vi "UVflourescence.vi"() -> ()   [LabVIEW 2009]
uses:
  <vilib>/DAQmx/write.llb/DAQmx Write (Digital Wfm 1Chan NSamp).vi
  <vilib>/DAQmx/configure/timing.llb/DAQmx Timing (Sample Clock).vi
  <vilib>/DAQmx/create/channels.llb/DAQmx Create Channel (DO-Digital Output).vi
  <vilib>/DAQmx/configure/timing.llb/DAQmx Timing (Implicit).vi
  <vilib>/DAQmx/create/channels.llb/DAQmx Create Channel (CO-Pulse Generation-Frequency).vi
  <vilib>/DAQmx/create/channels.llb/DAQmx Create Channel (CI-Count Edges).vi
  <vilib>/Waveform/DWDTOps.llb/DWDT Digital Size.vi
  <vilib>/DAQmx/read.llb/DAQmx Read (Counter 1D U32 1Chan NSamp).vi
  Program Files/National Instruments/LabVIEW 2009/resource/objmgr/daqmx.rc
  <vilib>/Analysis/NI_AALBase.lvlib
panel:
  out "Mean/Variance":dbl
  out "Variance":dbl format="%0.2f"
  out "Mean":dbl format="%0.2f"
  out "PMT Counts":cluster{"mean":dbl, u32}(graph)
  in  "Samples per block":i32=100 min=1 step=1
  out "x = 0?":bool
  out "Waveform Graph":u32[](graph)
  in  "Stop":bool
  in  "Sample Time":dbl=5e-07
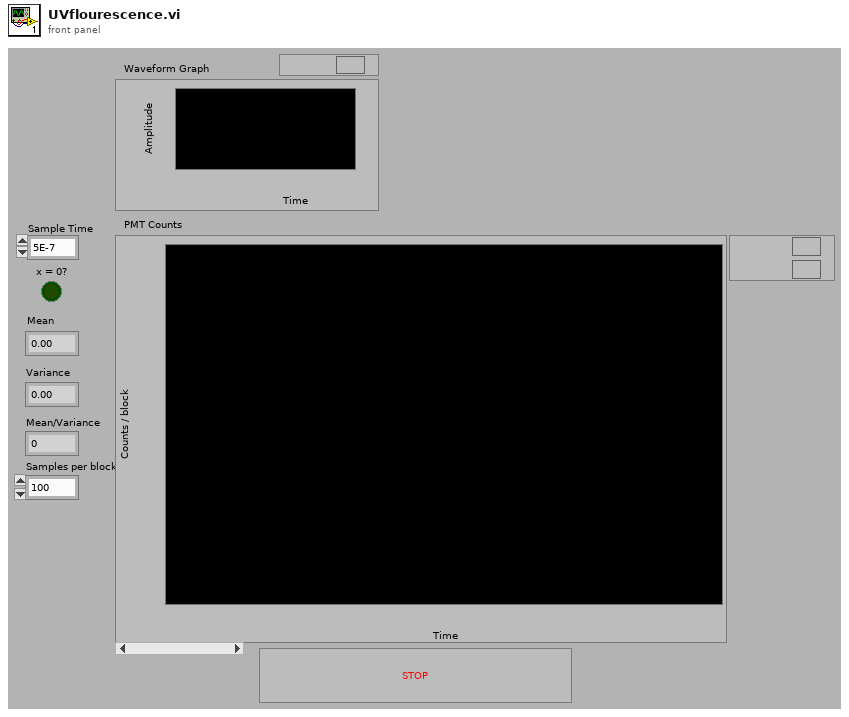
[diagram p1: front panel]
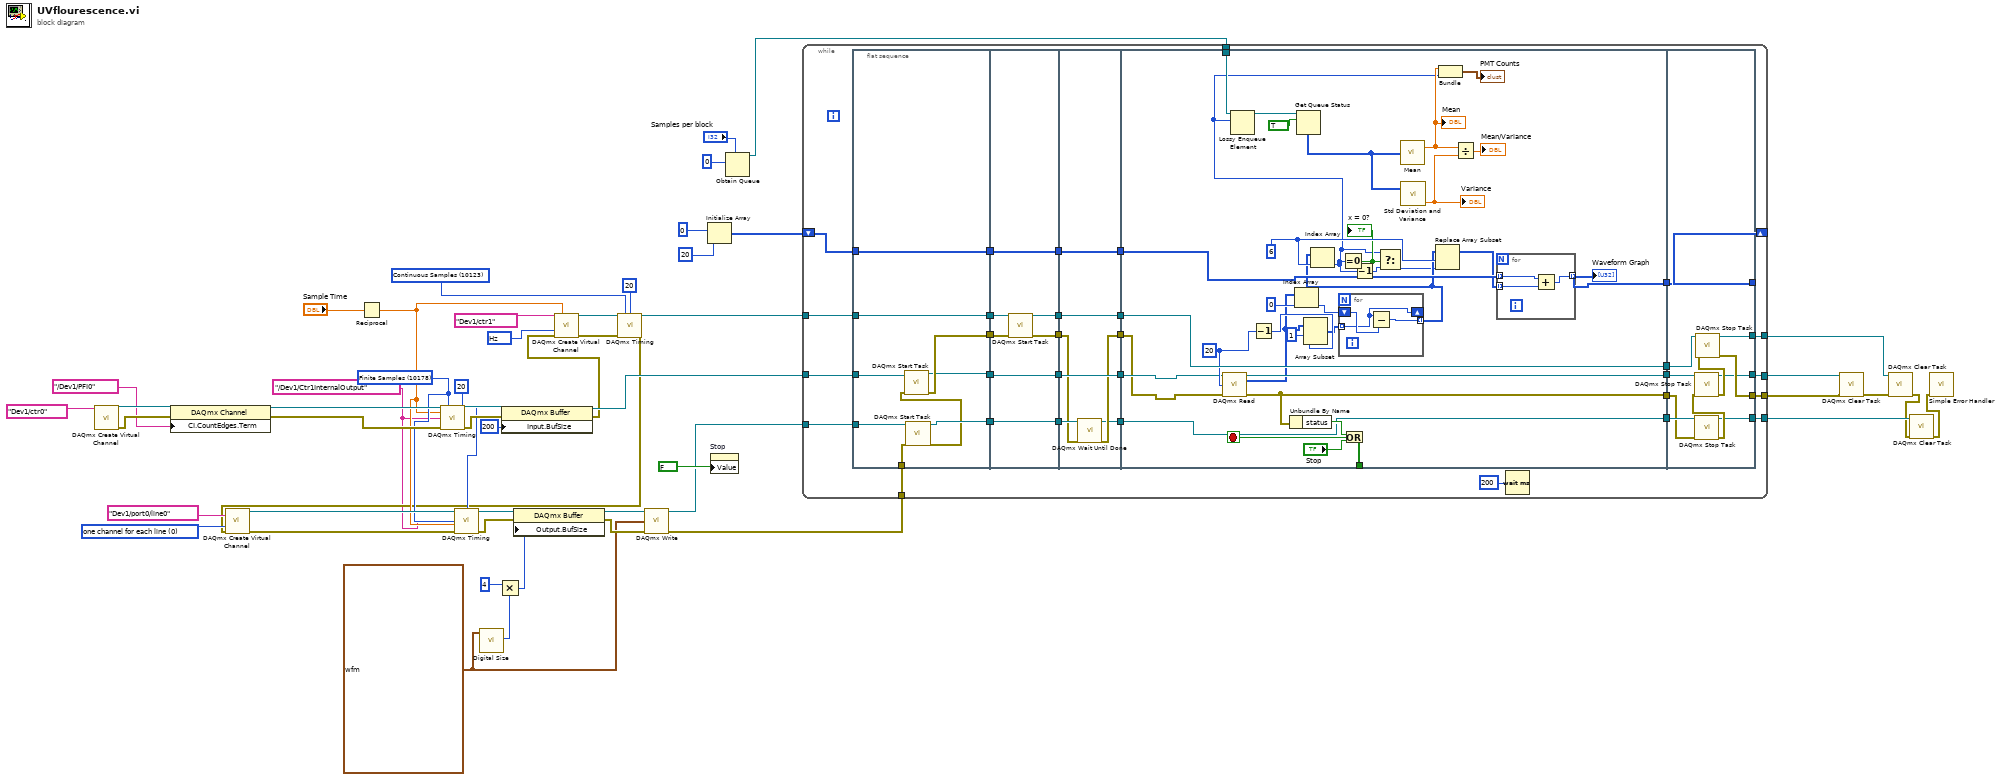
[diagram p0: block diagram]
diagram:
  w19 = digitalwaveform {"t0"=timestamp(0 s since 1904-01-01), "dt"=1e-06, "Y"={"transitions"=[], "data"=[[1], [1], [1], [1], [0], [0], [0], [0], [0], [1], [1], [1], [1], [0], [0], [0], [0], [0], [0], [0]]}, "error"={"status"=FALSE, "code"=37421928, "source"=""}} ("data")
  w24 = 0 items=["one channel for each line", "one channel for all lines"] ("line grouping")
  w14 = 10178 items=["Finite Samples"=10178, "Continuous Samples"=10123, "Hardware Timed Single Point"=12522] ("sample mode")
  w15 = 20 ("samples per channel")
  w4 = tag "/Dev1/Ctr1InternalOutput" ("source")
  w50 = 10373 items=["Hz"=10373] ("units")
  w42 = 10123 items=["Finite Samples"=10178, "Continuous Samples"=10123, "Hardware Timed Single Point"=12522] ("sample mode")
  n1 = call-poly <vilib>:"DAQmx Create Virtual Channel.vi"("counter"=tag "Dev1/ctr0") -> ("task out"=w47:refnum<k21>, "error out"=w46:errorcluster)  [unwired: 13 in]
  n2 = property class="DAQmx Channel"(reference=w47, error in=w46, "CI.CountEdges.Term"=tag "/Dev1/PFI0") -> (reference out=w37:refnum<k21>, error out=w38:errorcluster)
  n3 = Reciprocal(x="Sample Time") -> (1/x=w13:dbl)
  n4 = call-poly <vilib>:"DAQmx Timing.vi"("task/channels in"=w37, "sample mode"=w14, "samples per channel"=w15, "rate"=w13, "source"=w4, "error in"=w38) -> ("task out"=w31:refnum<k21>, "error out"=w30:errorcluster)  [unwired: 8 in]
  n5 = call-poly <vilib>:"Digital Size.vi"("digital waveform in"=w19) -> ("number of samples"=w18:i32)  [unwired: 7 in, 3 out]
  n6 = Multiply(x=4, y=w18) -> (x*y=w16:i32)
  n7 = property class="DAQmx Buffer"(reference=w31, error in=w30, "Input.BufSize"=u32 200) -> (reference out=w29:refnum<k21>, error out=w28:errorcluster)
  n8 = call-poly <vilib>:"DAQmx Create Virtual Channel.vi"("frequency"=w13, "counter"=tag "Dev1/ctr1", "units"=w50, "error in"=w28) -> ("task out"=w49:refnum<k21>, "error out"=w48:errorcluster)  [unwired: 10 in]
  n9 = call-poly <vilib>:"DAQmx Timing.vi"("task/channels in"=w49, "sample mode"=w42, "samples per channel"=20, "error in"=w48) -> ("task out"=w11:refnum<k21>, "error out"=w8:errorcluster)  [unwired: 10 in]
  n10 = call-poly <vilib>:"DAQmx Create Virtual Channel.vi"("lines"=tag "Dev1/port0/line0", "line grouping"=w24, "error in"=w8) -> ("task out"=w26:refnum<k21>, "error out"=w25:errorcluster)  [unwired: 11 in]
  n11 = call-poly <vilib>:"DAQmx Timing.vi"("task/channels in"=w26, "sample mode"=w14, "samples per channel"=w15, "rate"=w13, "source"=w4, "error in"=w25) -> ("task out"=w22:refnum<k21>, "error out"=w21:errorcluster)  [unwired: 8 in]
  n12 = property class="DAQmx Buffer"(reference=w22, error in=w21, "Output.BufSize"=w16) -> (reference out=w12:refnum<k21>, error out=w20:errorcluster)
  n13 = call-poly <vilib>:"DAQmx Write.vi"("task/channels in"=w12, "data"=w19, "error in"=w20) -> ("task out"=w10:refnum<k21>, "error out"=w9:errorcluster)  [unwired: 10 in, 1 out]
  n14 = Initialize Array(0, 20 ("dimension size")) -> (w39:i32[])
  n15 = property on="Stop" class="Bool (strict)"("Value"=FALSE) -> ()  [unwired: 2 in, 2 out]
  n16 = Obtain Queue(max queue size (-1, unlimited)="Samples per block", element data type=u32 0) -> (queue out=w1:refnum<queue>)  [unwired: 3 in, 2 out]
  n17 = while {
    tunnel: [w81] -> w34
    tunnel: [w82] -> w35
    tunnel: w29 -> [w83]
    shift-right: [w75] -> _
    shift-left: w39 -> [w84]
    tunnel: w11 -> [w80]
    tunnel: [w70] -> w33
    tunnel: w10 -> [w69]
    tunnel: w9 -> [w68]
    tunnel: [w55] -> w7
    tunnel: w1 -> [w53]
    stop <- w85 stop-if-true
    n18 = flat-sequence {
      tunnel: w80 -> [w93]
      tunnel: w83 -> [w92]
      tunnel: w84 -> [w94]
      tunnel: [w94] -> w79
      tunnel: [w90] -> w78
      tunnel: [w93] -> w77
      tunnel: [w91] -> w76
      tunnel: w69 -> [w89]
      tunnel: w68 -> [w88]
      tunnel: [w87] -> w58
      tunnel: [w101] -> w67
      tunnel: [w100] -> w65
      tunnel: w79 -> [w101]
      tunnel: w78 -> [w100]
      tunnel: w77 -> [w99]
      tunnel: w76 -> [w98]
      tunnel: [w97] -> w63
      tunnel: [w96] -> w61
      tunnel: [w95] -> w59
      tunnel: w58 -> [w95]
      tunnel: w67 -> [w108]
      tunnel: [w108] -> w66
      tunnel: w65 -> [w107]
      tunnel: [w107] -> w64
      tunnel: w63 -> [w106]
      tunnel: [w106] -> w62
      tunnel: w61 -> [w104]
      tunnel: [w103] -> w60
      tunnel: w59 -> [w105]
      tunnel: [w102] -> w56
      tunnel: [w141] -> w85
      tunnel: w66 -> [w128]
      tunnel: w64 -> [w126]
      tunnel: [w137] -> w74
      tunnel: [w136] -> w73
      tunnel: [w127] -> w72
      tunnel: [w138] -> w71
      tunnel: w62 -> [w138]
      tunnel: w60 -> [w125]
      tunnel: [w124] -> w57
      tunnel: w56 -> [w124]
      tunnel: w53 -> [w110]
      tunnel: [w158] -> w75
      tunnel: [w154] -> w81
      tunnel: [w153] -> w82
      tunnel: w74 -> [w156]
      tunnel: w73 -> [w150]
      tunnel: w72 -> [w158]
      tunnel: w71 -> [w157]
      tunnel: [w152] -> w70
      tunnel: w57 -> [w151]
      tunnel: [w148] -> w55
      frame #0 {
        n19 = call <vilib>:"DAQmx Start Task.vi"("task/channels in"=w89, "error in"=w88) -> ("task out"=w87:refnum<k21>, "error out"=w86:errorcluster)  [unwired: 12 in]
        n20 = call <vilib>:"DAQmx Start Task.vi"("task/channels in"=w92, "error in"=w86) -> ("task out"=w90:refnum<k21>, "error out"=w91:errorcluster)  [unwired: 12 in]
      }
      frame #1 {
        n21 = call <vilib>:"DAQmx Start Task.vi"("task/channels in"=w99, "error in"=w98) -> ("task out"=w97:refnum<k21>, "error out"=w96:errorcluster)  [unwired: 12 in]
      }
      frame #2 {
        n22 = call <vilib>:"DAQmx Wait Until Done.vi"("task/channels in"=w105, "error in"=w104) -> ("task out"=w102:refnum<k21>, "error out"=w103:errorcluster)  [unwired: 12 in]
      }
      frame #3 {
        w123 = 6 ("index")
        w130 = 20 ("number of samples per channel")
        n23 = call-poly <vilib>:"DAQmx Read.vi"("task/channels in"=w126, "number of samples per channel"=w130, "error in"=w125) -> ("task out"=w137:refnum<k21>, "data"=w129:u32[], "error out"=w136:errorcluster)  [unwired: 10 in]
        n24 = Decrement(x=w130) -> (x-1=w132:i32)
        n25 = Unbundle By Name(w136) -> ("status"=w140:bool)
        n26 = Index Array(array=w129, index=0) -> (element=w134:u32)
        n27 = Array Subset(array=w129, index=1, length=w132) -> (w131:u32[])
        n28 = for {
          tunnel: [w147] -> w122 mode=indexing
          shift-right: [w145] -> _
          shift-left: w134 -> [w146]
          tunnel: w131 -> [w145] mode=indexing
          n29 = Subtract(x=w145, y=w146) -> (x-y=w147:u32)
        }
        n30 = Index Array(array=w122, index=w123) -> (element=w109:u32)
        n31 = Lossy Enqueue Element(queue=w110, element=w109) -> (queue out=w117:refnum<queue>)  [unwired: 1 in, 3 out]
        n32 = Get Queue Status(queue=w117, return elements? (F)=TRUE) -> (elements=w115:u32[])  [unwired: 1 in, 7 out]
        n33 = Equal To 0?(x=w109) -> (x = 0?=w120:bool)
        "x = 0?" <- w120
        n34 = Or(x=w140, y="Stop") -> (x .or. y?=w141:bool)
        n35 = Decrement(x=w109) -> (x-1=w119:u32)
        n36 = Select(t=w109, s=w120, f=w119) -> (s? t:f=w118:u32)
        n37 = call <vilib>:"Mean.vi"("X"=w115) -> ("mean"=w111:dbl)  [unwired: 1 out]
        "Mean" <- w111
        n38 = call <vilib>:"Std Deviation and Variance.vi"("X"=w115) -> ("variance"=w114:dbl)  [unwired: 1 in, 2 out]
        "Variance" <- w114
        n39 = Replace Array Subset(array=w122, new element=w118, index=w123) -> (w121:u32[])
        n40 = Bundle("mean"=w111, w109) -> (→"PMT Counts":cluster{"mean":dbl, u32})  [unwired: 1 in]
        n41 = Divide(x=w111, y=w114) -> (x/y=→"Mean/Variance":dbl)
        n42 = for {
          tunnel: w128 -> [w144] mode=indexing
          tunnel: w121 -> [w143] mode=indexing
          tunnel: [w142] -> w127 mode=indexing
          n43 = Add(x=w144, y=w143) -> (x+y=w142:u32)
        }
        "Waveform Graph" <- w127
      }
      frame #4 {
        n44 = call <vilib>:"DAQmx Stop Task.vi"("task/channels in"=w151, "error in"=w150) -> ("task out"=w148:refnum<k21>, "error out"=w149:errorcluster)  [unwired: 12 in]
        n45 = call <vilib>:"DAQmx Stop Task.vi"("task/channels in"=w156, "error in"=w149) -> ("task out"=w153:refnum<k21>, "error out"=w155:errorcluster)  [unwired: 12 in]
        n46 = call <vilib>:"DAQmx Stop Task.vi"("task/channels in"=w157, "error in"=w155) -> ("task out"=w152:refnum<k21>, "error out"=w154:errorcluster)  [unwired: 12 in]
      }
    }
    n47 = Wait (ms)(milliseconds to wait=u32 200) -> ()  [unwired: 1 out]
  }
  n48 = call <vilib>:"DAQmx Clear Task.vi"("task in"=w35, "error in"=w34) -> ("error out"=w44:errorcluster)  [unwired: 13 in]
  n49 = call <vilib>:"DAQmx Clear Task.vi"("task in"=w33, "error in"=w44) -> ("error out"=w6:errorcluster)  [unwired: 13 in]
  n50 = call <vilib>:"DAQmx Clear Task.vi"("task in"=w7, "error in"=w6) -> ("error out"=w5:errorcluster)  [unwired: 13 in]
  n51 = call <vilib>:"Simple Error Handler.vi"("error in (no error)"=w5) -> ()  [unwired: 4 in, 5 out]
